vi "GetTemperature.vi"(11 "packet in":u8[](array[numeric])) -> (3 "temperature (degC)":dbl)   [LabVIEW 2018]
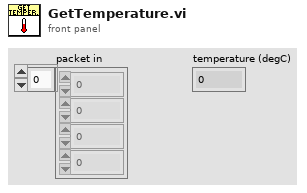
[diagram p1: front panel]
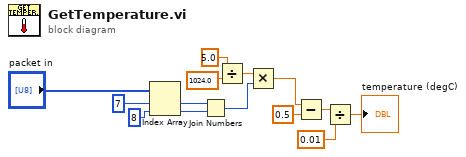
[diagram p0: block diagram]
diagram:
  n1 = Index Array(array="packet in", index #1=7 ("index"), index #2=8 ("index")) -> (element #1=w4:u8, element #2=w3:u8)
  n2 = Join Numbers(hi=w4, lo=w3) -> ((hi.lo)=w13:u16)
  n3 = Divide(x=5.0, y=1024.0 ("x")) -> (x/y=w12:dbl)
  n4 = Multiply(x=w12, y=w13) -> (x*y=w14:dbl)
  n5 = Subtract(x=w14, y=0.5) -> (x-y=w9:dbl)
  n6 = Divide(x=w9, y=0.01) -> (x/y=→"temperature (degC)":dbl)
